vi "ReadExpectedDependencies.vi"(8 "error in (no error)":errorcluster, 11 "Library Name":string) -> (0 "error out":errorcluster, 1 "ExpectedDeps Path":path, 2 "Expected Indirect Dependencies":string[](array[string]), 3 "Expected Direct Dependencies":string[](array[string]), 5 "Found?":bool)   [LabVIEW 2019, in "DepsWatch.lvlib"]
uses:
  DepsWatch.lvlib
  <vilib>/Utility/config.llb/NI_LVConfig.lvlib
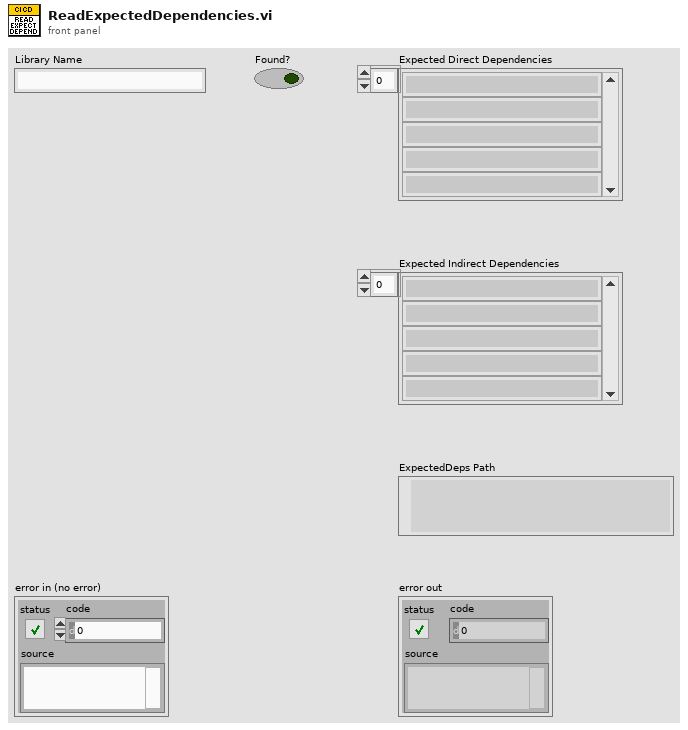
[diagram p1: front panel]
types:
  T1 = typedef "NI_LVConfig.lvlib/Config Data RefNum.ctl" = refnum<k1>
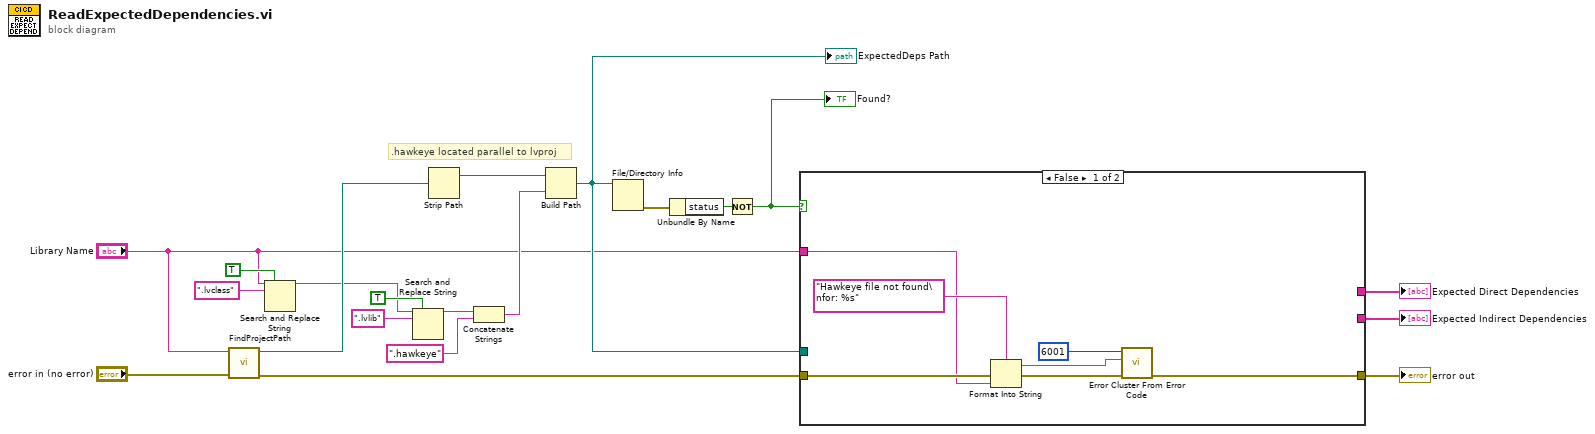
[diagram p0: block diagram]
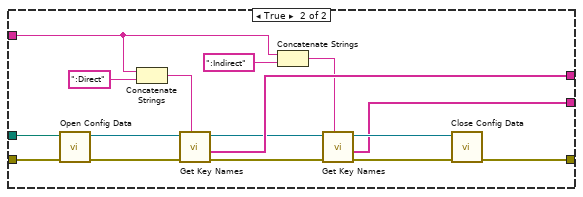
[diagram p2: hidden frame]
diagram:
  # ".hawkeye located parallel to lvproj"
  n1 = call "FindProjectPath.vi"("error in (no error)"="error in (no error)", "Library/Class Name"="Library Name") -> ("error out"=w12:errorcluster, "Project Path"=w19:path)  [unwired: 7 in, 1 out]
  n2 = Search and Replace String(replace all?=TRUE ("replace all? (F)"), input string="Library Name", search string=".lvclass") -> (result string=w3:string)  [unwired: 5 in, 3 out]
  n3 = Search and Replace String(replace all?=TRUE ("replace all? (F)"), input string=w3, search string=".lvlib") -> (result string=w15:string)  [unwired: 5 in, 3 out]
  n4 = Strip Path(path=w19) -> (stripped path=w18:path)  [unwired: 1 out]
  n5 = Concatenate Strings(w15, ".hawkeye" ("string")) -> (w13:string)
  n6 = Build Path(base path=w18, name or relative path=w13) -> (appended path=w9:path)
  "ExpectedDeps Path" <- w9
  n7 = File/Directory Info(path=w9) -> (error out=w6:errorcluster)  [unwired: 1 in, 6 out]
  n8 = Unbundle By Name(w6) -> ("status"=w7:bool)
  n9 = Not(x=w7) -> (.not. x?=w8:bool)
  "Found?" <- w8
  n10 = case shown="False" w8 {
    tunnel: w12 -> [w26 w43]
    tunnel: "Library Name" -> [w24 w28]
    tunnel: [w21 w38] -> w11
    tunnel: w9 -> [_ w42]
    tunnel: [_ w39] -> w10
    tunnel: [_ w30] -> w1
    frame False {
      n11 = Format Into String(format string="Hawkeye file not found\nfor: %s" ("error message (\"\")"), error in=w26, w24) -> (resulting string=w23:string, error out=w22:errorcluster)  [unwired: 1 in]
      n12 = call <vilib>:"Error Cluster From Error Code.vi"("error in (no error)"=w22, "error message (\"\")"=w23, "error code (0)"=6001) -> ("error out"=w21:errorcluster)  [unwired: 6 in]
    }
    frame True {
      n13 = call <vilib>:"Open Config Data.vi"("error in (no error)"=w43, "configuration file path"=w42) -> ("error out"=w41:errorcluster, "refnum"=w40:T1)  [unwired: 7 in, 1 out]
      n14 = Concatenate Strings(w28, ":Direct" ("string")) -> (w29:string)
      n15 = call <vilib>:"Get Key Names.vi"("section"=w29, "error in (no error)"=w41, "refnum"=w40) -> ("error out"=w33:errorcluster, "key names"=w39:string[], "refnum out"=w35:T1)  [unwired: 5 in, 1 out]
      n16 = Concatenate Strings(w28, ":Indirect" ("string")) -> (w31:string)
      n17 = call <vilib>:"Get Key Names.vi"("section"=w31, "error in (no error)"=w33, "refnum"=w35) -> ("error out"=w32:errorcluster, "key names"=w30:string[], "refnum out"=w34:T1)  [unwired: 5 in, 1 out]
      n18 = call <vilib>:"Close Config Data.vi"("error in (no error)"=w32, "refnum"=w34) -> ("error out"=w38:errorcluster)  [unwired: 8 in, 1 out]
    }
  }
  "error out" <- w11
  "Expected Direct Dependencies" <- w10
  "Expected Indirect Dependencies" <- w1
